vi "SIM comprehensive manager (for core).vi"(3 "Simulation data":T1={"continuous integrator"=enum."RK 1 (Euler)", "initial time"=0.0, "final time"=0.0, "step size"=0.0, "proposed step size"=0.0, "max step size"=0.0, "min step size"=0.0, "discrete time step"=0.0, "max step ratio"=0.0, "Diag Eval Stage"=enum."Init", "Substep Index"=0, "Timestep Index"=0.0, "simulation time"=0.0, "current timestep base"=0.0, "proposed step time"=0.0, "absolute tolerance"=0.0, "relative tolerance"=0.0, "step accepted?"=FALSE, "step complete?"=FALSE, "Halt?"=FALSE, "reset integrator?"=FALSE, "machine epsilon"=0.0, "min float"=0.0, "error"={"status"=FALSE, "code"=0, "source"=""}, "Method Order"=0, "Finished Late [i-1]"=FALSE, "Discrete step?"=FALSE, "NaN and Inf check?"=FALSE, "Final Timestep Index"=0.0, "(maj+disc)or(init)?"=FALSE, "Full Solver Reset"=TRUE, "Execution Mode"=enum."Simulate to Completion", "check vector sizes?"=FALSE, "solver handles zc?"=FALSE, "Simulation Registry"={"Current Idx"=0, "Node Tags"=[], "Node Headers"=[], "Node Data"=[], "Cont State data"={"inputs"=[], "outputs"=[], "reset"=[], "lower limits"=[], "upper limits"=[], "limit types"=[], "reset types"=[], "initial conditions"=[], "reset I.C."=[], "limited?"=[], "State Names"=[]}, "DiscreteInfo"={"tick period (sec)"=0.0, "time (ticks)"=0, "fire?"=[], "registry"={"period (sec)"=[], "skew (sec)"=[], "period (tick)"=[], "skew (tick)"=[]}, "discrete \nblocks?"=FALSE, "steps per tick"=0.0, "steps to tick"=0.0, "discrete \ntick?"=FALSE}, "Disc State data"={"Disc States"=[], "State Names"=[]}, "Registry Error"={"Error Block ID"=0, "code"=0}, "ZC Indices"=[]}, "variable step solver?"=FALSE, "First Substep?"=FALSE, "Continuous States?"=FALSE} {"min float" format="%.1e"; "proposed step size" format="%.1e"; "proposed step time" format="%.1e"; "max step ratio" format="%.1e"; "min step size" format="%.1e"; "machine epsilon" format="%.1e"; "discrete time step" format="%.1e"; "max step size" format="%.1e"; "current timestep base" format="%.1e"; "final time" format="%.1e"; "simulation time" format="%.1e"; "relative tolerance" format="%.1e"; "absolute tolerance" format="%.1e"; "Substep Index" format="%.1e"; "step size" format="%.1e"; "initial time" format="%.1e"}) -> (0 "step complete?":bool, 1 "Simulation data out":T1={"continuous integrator"=enum."RK 1 (Euler)", "initial time"=0.0, "final time"=0.0, "step size"=0.0, "proposed step size"=0.0, "max step size"=0.0, "min step size"=0.0, "discrete time step"=0.0, "max step ratio"=0.0, "Diag Eval Stage"=enum."Init", "Substep Index"=0, "Timestep Index"=0.0, "simulation time"=0.0, "current timestep base"=0.0, "proposed step time"=0.0, "absolute tolerance"=0.0, "relative tolerance"=0.0, "step accepted?"=FALSE, "step complete?"=FALSE, "Halt?"=FALSE, "reset integrator?"=FALSE, "machine epsilon"=0.0, "min float"=0.0, "error"={"status"=FALSE, "code"=0, "source"=""}, "Method Order"=0, "Finished Late [i-1]"=FALSE, "Discrete step?"=FALSE, "NaN and Inf check?"=FALSE, "Final Timestep Index"=0.0, "(maj+disc)or(init)?"=FALSE, "Full Solver Reset"=TRUE, "Execution Mode"=enum."Simulate to Completion", "check vector sizes?"=FALSE, "solver handles zc?"=FALSE, "Simulation Registry"={"Current Idx"=0, "Node Tags"=[], "Node Headers"=[], "Node Data"=[], "Cont State data"={"inputs"=[], "outputs"=[], "reset"=[], "lower limits"=[], "upper limits"=[], "limit types"=[], "reset types"=[], "initial conditions"=[], "reset I.C."=[], "limited?"=[], "State Names"=[]}, "DiscreteInfo"={"tick period (sec)"=0.0, "time (ticks)"=0, "fire?"=[], "registry"={"period (sec)"=[], "skew (sec)"=[], "period (tick)"=[], "skew (tick)"=[]}, "discrete \nblocks?"=FALSE, "steps per tick"=0.0, "steps to tick"=0.0, "discrete \ntick?"=FALSE}, "Disc State data"={"Disc States"=[], "State Names"=[]}, "Registry Error"={"Error Block ID"=0, "code"=0}, "ZC Indices"=[]}, "variable step solver?"=FALSE, "First Substep?"=FALSE, "Continuous States?"=FALSE} {"min float" format="%.1e"; "proposed step size" format="%.1e"; "proposed step time" format="%.1e"; "max step ratio" format="%.1e"; "min step size" format="%.1e"; "machine epsilon" format="%.1e"; "discrete time step" format="%.1e"; "max step size" format="%.1e"; "current timestep base" format="%.1e"; "final time" format="%.1e"; "simulation time" format="%.1e"; "relative tolerance" format="%.1e"; "absolute tolerance" format="%.1e"; "Substep Index" format="%.1e"; "step size" format="%.1e"; "initial time" format="%.1e"})   [LabVIEW 2017]
uses:
  SIM simulation data.ctl
  SIM integration method.ctl
  SIM diagram eval stage.ctl
  SIMSCR Execution Mode.ctl
  SIM Simulation Registry.ctl
  SIM Registry Node Header.ctl
  SIM Registry Node Record.ctl
  SIM trigger type.ctl
  SIM solver state data.ctl
  SIM limit type.ctl
  SIM discrete data.ctl
  SIM Discrete state data.ctl
  SIM Simulation Registry Error.ctl
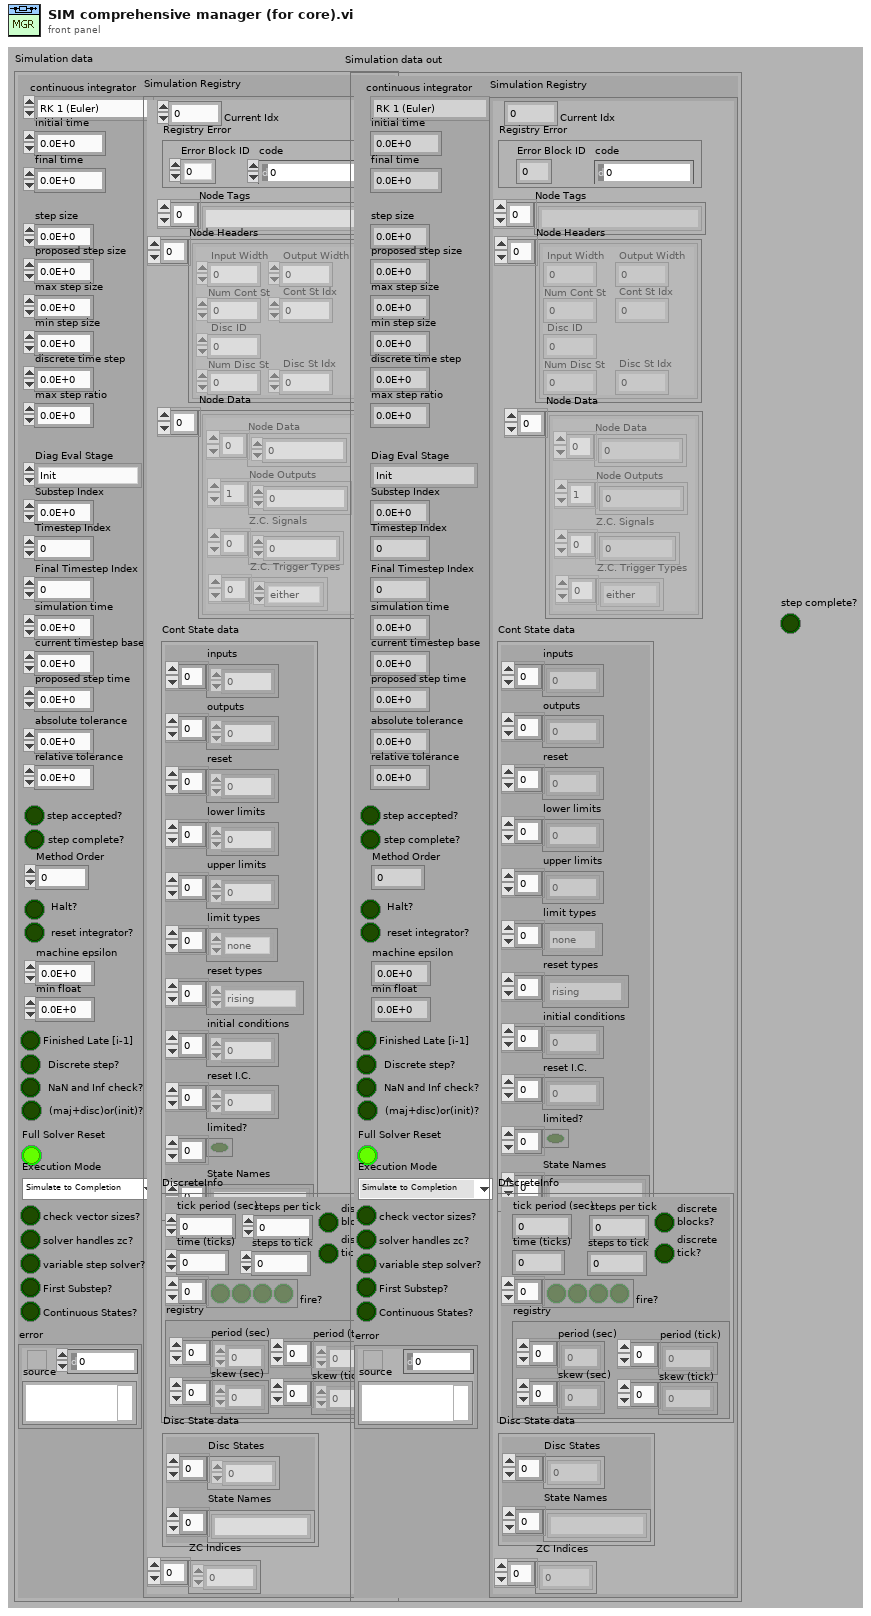
[diagram p1: front panel]
types:
  T1 = typedef "SIM simulation data.ctl" = cluster{"continuous integrator":T2, "initial time":dbl, "final time":dbl, "step size":dbl, "proposed step size":dbl, "max step size":dbl, "min step size":dbl, "discrete time step":dbl, "max step ratio":dbl, "Diag Eval Stage":T3, "Substep Index":i32, "Timestep Index":dbl, "simulation time":dbl, "current timestep base":dbl, "proposed step time":dbl, "absolute tolerance":dbl, "relative tolerance":dbl, "step accepted?":bool, "step complete?":bool, "Halt?":bool, "reset integrator?":bool, "machine epsilon":dbl, "min float":dbl, "error":errorcluster, "Method Order":u32, "Finished Late [i-1]":bool, "Discrete step?":bool, "NaN and Inf check?":bool, "Final Timestep Index":dbl, "(maj+disc)or(init)?":bool, "Full Solver Reset":bool, "Execution Mode":T4, "check vector sizes?":bool, "solver handles zc?":bool, "Simulation Registry":T5, "variable step solver?":bool, "First Substep?":bool, "Continuous States?":bool}
  T2 = typedef "SIM integration method.ctl" = enum16{"RK 1 (Euler)", "Linearizer", "State Query", "Trim Eval", "Adams", "RK 3", "RK 4", "RK 45", "BDF", "RK 2", "RK 23", "Rosenbrock", "Discrete States Only"}
  T3 = typedef "SIM diagram eval stage.ctl" = enum16{"Init", "Minor Substep", "Major Substep", "Final"}
  T4 = typedef "SIMSCR Execution Mode.ctl" = enum16{"Simulate to Completion", "Single Time-Step Simulation (Fixed Step Only)"}
  T5 = typedef "SIM Simulation Registry.ctl" = cluster{"Current Idx":i32, "Node Tags":string[], "Node Headers":T6[], "Node Data":T7[], "Cont State data":T9, "DiscreteInfo":T11, "Disc State data":T12, "Registry Error":T13, "ZC Indices":i32[]}
  T6 = typedef "SIM Registry Node Header.ctl" = cluster{"Input Width":i32, "Disc ID":i32, "Num Cont St":i32, "Cont St Idx":i32, "Num Disc St":i32, "Disc St Idx":i32, "Output Width":i32}
  T7 = typedef "SIM Registry Node Record.ctl" = cluster{"Node Data":dbl[], "Node Outputs":dbl[], "Z.C. Signals":dbl[], "Z.C. Trigger Types":T8[]}
  T8 = typedef "SIM trigger type.ctl" = enum16{"rising", "falling", "either", "none"}
  T9 = typedef "SIM solver state data.ctl" = cluster{"inputs":dbl[], "outputs":dbl[], "reset":dbl[], "lower limits":dbl[], "upper limits":dbl[], "limit types":T10[], "reset types":T8[], "initial conditions":dbl[], "reset I.C.":dbl[], "limited?":bool[], "State Names":string[]}
  T10 = typedef "SIM limit type.ctl" = enum16{"upper", "lower", "both", "none"}
  T11 = typedef "SIM discrete data.ctl" = cluster{"tick period (sec)":dbl, "time (ticks)":i32, "fire?":bool[], "registry":cluster{"period (sec)":dbl[], "skew (sec)":dbl[], "period (tick)":i32[], "skew (tick)":i32[]}, "discrete \nblocks?":bool, "steps per tick":dbl, "steps to tick":dbl, "discrete \ntick?":bool}
  T12 = typedef "SIM Discrete state data.ctl" = cluster{"Disc States":dbl[], "State Names":string[]}
  T13 = typedef "SIM Simulation Registry Error.ctl" = cluster{"Error Block ID":i32, "code":i32}
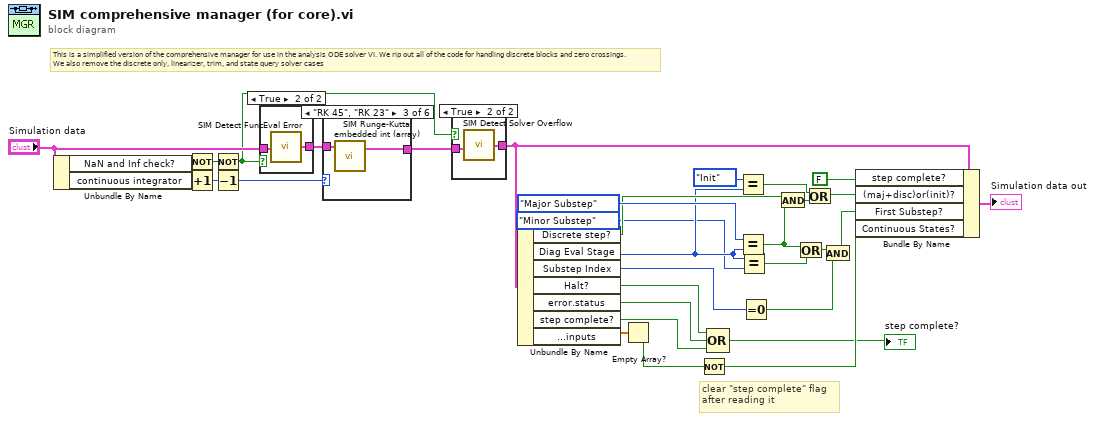
[diagram p0: block diagram]
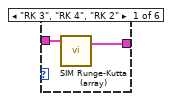
[diagram p2: hidden frame]
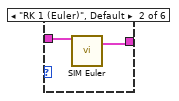
[diagram p3: hidden frame]
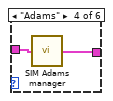
[diagram p4: hidden frame]
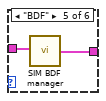
[diagram p5: hidden frame]
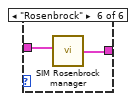
[diagram p6: hidden frame]
diagram:
  # "This is a simplified version of the comprehensive manager for use in the analysis ODE solver VI. We rip out all of the code for handling discrete blocks and zero crossings.\nWe also remove the discrete only, linearizer, trim, and state query solver cases"
  # "clear \"step complete\" flag\nafter reading it"
  n1 = Unbundle By Name("Simulation data") -> ("NaN and Inf check?"=w32:bool, "continuous integrator"=w33:T2)
  n2 = Not(x=w32) -> (.not. x?=w22:bool)
  n3 = Increment(x=w33) -> (x+1=w21:T2)
  n4 = Not(x=w22) -> (.not. x?=w1:bool)
  n5 = Decrement(x=w21) -> (x-1=w19:T2)
  n6 = case shown="True" w1 {
    tunnel: [w34 w36] -> w3
    tunnel: "Simulation data" -> [w34 w35]
    frame False {
    }
    frame True {
      n7 = call "SIM Detect FuncEval Error.vi"("Simulation data"=w35) -> ("Simulation data out"=w36:T1)
    }
  }
  n8 = case shown="\"RK 45\", \"RK 23\"" w19 {
    tunnel: w3 -> [w37 w40 w42 w44 w46 w48]
    tunnel: [w38 w39 w41 w43 w45 w47] -> w23
    frame "RK 3", "RK 4", "RK 2" {
      n9 = call "SIM Runge-Kutta (array).vi"("Simulation data"=w37) -> ("Simulation data out"=w38:T1)  [unwired: 1 in, 1 out]
    }
    frame "RK 1 (Euler)", Default {
      n10 = call "SIM Euler.vi"("Simulation data"=w40) -> ("Simulation data out"=w39:T1)  [unwired: 2 out]
    }
    frame "RK 45", "RK 23" {
      n11 = call "SIM Runge-Kutta embedded int (array).vi"("Simulation data"=w42) -> ("Simulation data out"=w41:T1)  [unwired: 2 out]
    }
    frame "Adams" {
      n12 = call "SIM Adams manager.vi"("Simulation data"=w44) -> ("Simulation data out"=w43:T1)
    }
    frame "BDF" {
      n13 = call "SIM BDF manager.vi"("Simulation data"=w46) -> ("Simulation data out"=w45:T1)
    }
    frame "Rosenbrock" {
      n14 = call "SIM Rosenbrock manager.vi"("Simulation data"=w48) -> ("Simulation data out"=w47:T1)
    }
  }
  n15 = case shown="True" w1 {
    tunnel: w23 -> [w49 w51]
    tunnel: [w49 w50] -> w2
    frame False {
    }
    frame True {
      n16 = call "SIM Detect Solver Overflow.vi"("Simulation data"=w51) -> ("Simulation data out"=w50:T1)
    }
  }
  n17 = Unbundle By Name(w2) -> ("Discrete step?"=w18:bool, "Diag Eval Stage"=w16:T3, "Substep Index"=w17:i32, "Halt?"=w24:bool, "error.status"=w25:bool, "step complete?"=w26:bool, "Simulation Registry.Cont State data.inputs"=w9:dbl[])
  n18 = Empty Array?(array=w9) -> (empty?=w8:bool)
  n19 = Not(x=w8) -> (.not. x?=w7:bool)
  n20 = Compound Arithmetic op=OR(w24, w25, w26) -> (→"step complete?":bool)
  n21 = Equal?(x=SIM_diagram_eval_stage."Init", y=w16) -> (x = y?=w31:bool)
  n22 = Equal?(x=SIM_diagram_eval_stage."Major Substep", y=w16) -> (x = y?=w14:bool)
  n23 = Equal?(x=w16, y=SIM_diagram_eval_stage."Minor Substep" ("x")) -> (x = y?=w13:bool)
  n24 = Equal To 0?(x=w17) -> (x = 0?=w11:bool)
  n25 = And(x=w18, y=w14) -> (x .and. y?=w28:bool)
  n26 = Or(x=w14, y=w13) -> (x .or. y?=w10:bool)
  n27 = Or(x=w31, y=w28) -> (x .or. y?=w20:bool)
  n28 = And(x=w10, y=w11) -> (x .and. y?=w12:bool)
  n29 = Bundle By Name(cluster=w2, "step complete?"=FALSE, "(maj+disc)or(init)?"=w20, "First Substep?"=w12, "Continuous States?"=w7) -> (→"Simulation data out":T1)
